vi "Save Test Info.vi"   [LabVIEW 2017]
uses:
  <vilib>/Utility/config.llb/Write Key (String).vi
  <vilib>/Utility/config.llb/NI_LVConfig.lvlib
types:
  T1 = typedef "NI_LVConfig.lvlib/Config Data RefNum.ctl" = refnum<k1>
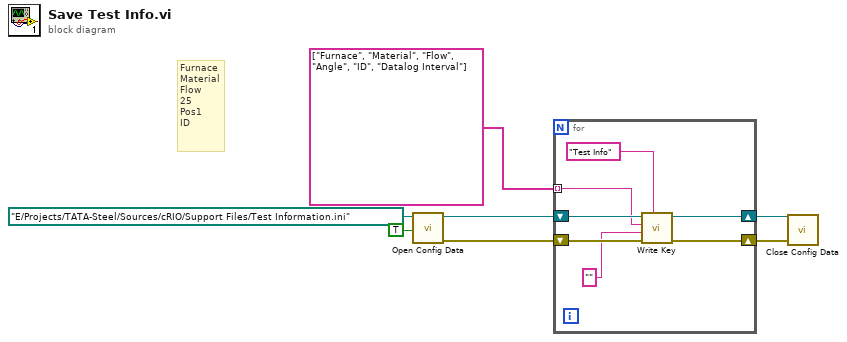
[diagram p0: block diagram]
diagram:
  # "Furnace\nMaterial\nFlow\n25\nPos1\nID"
  n1 = call <vilib>:"Open Config Data.vi"("create file if necessary (T)"=TRUE, "configuration file path"=path "E:/Projects/TATA-Steel/Sources/cRIO/Support Files/Test Information.ini") -> ("error out"=w5:errorcluster, "refnum"=w7:T1)  [unwired: 7 in, 1 out]
  n2 = for {
    shift-right: [w13] -> w6
    shift-left: w7 -> [w14]
    shift-right: [w11] -> w4
    shift-left: w5 -> [w12]
    tunnel: string[] ["Furnace", "Material", "Flow", "Angle", "ID", "Datalog Interval"] ("section") -> [w10] mode=indexing
    n3 = call-poly <vilib>:"Write Key.vi"("section"="Test Info", "error in (no error)"=w12, "value"="" ("default value"), "key"=w10, "refnum"=w14) -> ("error out"=w11:errorcluster, "refnum out"=w13:T1)  [unwired: 4 in, 1 out]
  }
  n4 = call <vilib>:"Close Config Data.vi"("error in (no error)"=w4, "refnum"=w6) -> ()  [unwired: 8 in, 2 out]
